vi "extract states.vi"(11 "state":u16) -> (1 "pulse not yet sent":bool, 2 "next output":bool, 3 "current output":bool, 4 "counter index":u8)   [LabVIEW 2018, in "trigger-out.lvlib"]
uses:
  trigger-out.lvlib
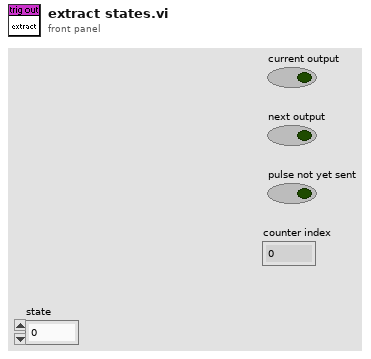
[diagram p1: front panel]
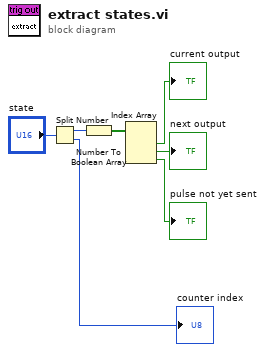
[diagram p0: block diagram]
diagram:
  n1 = Split Number(x="state") -> (hi(x)=w5:u8, lo(x)=→"counter index":u8)
  n2 = Number To Boolean Array(number=w5) -> (Boolean array=w4:bool[])
  n3 = Index Array(array=w4) -> (element #1=→"current output":bool, element #2=→"next output":bool, element #3=→"pulse not yet sent":bool)  [unwired: 3 in]
